vi "Camera Open.vi"(10 "Cluster":T1={"VideoMode"=81, "Brightness"=-1, "Sharpness"=-1, "White Balance"=-1, "Saturation"=-1, "Exposure"=-1} {"VideoMode" items=["640 x 480 YUY 2 30.00 fps", "640 x 480 YUY 2 20.00 fps", "640 x 480 YUY 2 15.00 fps", "640 x 480 YUY 2 10.00 fps", "640 x 480 YUY 2 7.50 fps", "1280 x 720 YUY 2 10.00 fps", "1280 x 720 YUY 2 7.50 fps", "960 x 544 YUY 2 15.00 fps", "960 x 544 YUY 2 10.00 fps", "960 x 544 YUY 2 7.50 fps", "800 x 448 YUY 2 20.00 fps", "800 x 448 YUY 2 15.00 fps", "800 x 448 YUY 2 10.00 fps", "800 x 448 YUY 2 7.50 fps", "640 x 360 YUY 2 30.00 fps", "640 x 360 YUY 2 20.00 fps", "640 x 360 YUY 2 15.00 fps", "640 x 360 YUY 2 10.00 fps", "640 x 360 YUY 2 7.50 fps", "424 x 240 YUY 2 30.00 fps", "424 x 240 YUY 2 20.00 fps", "424 x 240 YUY 2 15.00 fps", "424 x 240 YUY 2 10.00 fps", "424 x 240 YUY 2 7.50 fps", "352 x 288 YUY 2 30.00 fps", "352 x 288 YUY 2 20.00 fps", "352 x 288 YUY 2 15.00 fps", "352 x 288 YUY 2 10.00 fps", "352 x 288 YUY 2 7.50 fps", "320 x 240 YUY 2 30.00 fps", "320 x 240 YUY 2 20.00 fps", "320 x 240 YUY 2 15.00 fps", "320 x 240 YUY 2 10.00 fps", "320 x 240 YUY 2 7.50 fps", "800 x 600 YUY 2 15.00 fps", "800 x 600 YUY 2 10.00 fps", "800 x 600 YUY 2 7.50 fps", "176 x 144 YUY 2 30.00 fps", "176 x 144 YUY 2 20.00 fps", "176 x 144 YUY 2 15.00 fps", "176 x 144 YUY 2 10.00 fps", "176 x 144 YUY 2 7.50 fps", "160 x 120 YUY 2 30.00 fps", "160 x 120 YUY 2 20.00 fps", "160 x 120 YUY 2 15.00 fps", "160 x 120 YUY 2 10.00 fps", "160 x 120 YUY 2 7.50 fps", "1280 x 800 YUY 2 10.00 fps", "640 x 480 JPEG 30.00 fps", "640 x 480 JPEG 20.00 fps", "640 x 480 JPEG 15.00 fps", "640 x 480 JPEG 10.00 fps", "640 x 480 JPEG 7.50 fps", "1280 x 720 JPEG 30.00 fps", "1280 x 720 JPEG 20.00 fps", "1280 x 720 JPEG 15.00 fps", "1280 x 720 JPEG 10.00 fps", "1280 x 720 JPEG 7.50 fps", "960 x 544 JPEG 30.00 fps", "960 x 544 JPEG 20.00 fps", "960 x 544 JPEG 15.00 fps", "960 x 544 JPEG 10.00 fps", "960 x 544 JPEG 7.50 fps", "800 x 448 JPEG 30.00 fps", "800 x 448 JPEG 20.00 fps", "800 x 448 JPEG 15.00 fps", "800 x 448 JPEG 10.00 fps", "800 x 448 JPEG 7.50 fps", "640 x 360 JPEG 30.00 fps", "640 x 360 JPEG 20.00 fps", "640 x 360 JPEG 15.00 fps", "640 x 360 JPEG 10.00 fps", "640 x 360 JPEG 7.50 fps", "800 x 600 JPEG 30.00 fps", "800 x 600 JPEG 20.00 fps", "800 x 600 JPEG 15.00 fps", "800 x 600 JPEG 10.00 fps", "800 x 600 JPEG 7.50 fps", "416 x 240 JPEG 30.00 fps", "416 x 240 JPEG 20.00 fps", "416 x 240 JPEG 15.00 fps", "416 x 240 JPEG 10.00 fps", "416 x 240 JPEG 7.50 fps", "352 x 288 JPEG 30.00 fps", "352 x 288 JPEG 20.00 fps", "352 x 288 JPEG 15.00 fps", "352 x 288 JPEG 10.00 fps", "352 x 288 JPEG 7.50 fps", "176 x 144 JPEG 30.00 fps", "176 x 144 JPEG 20.00 fps", "176 x 144 JPEG 15.00 fps", "176 x 144 JPEG 10.00 fps", "176 x 144 JPEG 7.50 fps", "320 x 240 JPEG 30.00 fps", "320 x 240 JPEG 20.00 fps", "320 x 240 JPEG 15.00 fps", "320 x 240 JPEG 10.00 fps", "320 x 240 JPEG 7.50 fps", "160 x 120 JPEG 30.00 fps", "160 x 120 JPEG 20.00 fps", "160 x 120 JPEG 15.00 fps", "160 x 120 JPEG 10.00 fps", "160 x 120 JPEG 7.50 fps"]}, 11 "InterfaceName":string) -> (0 "error out":errorcluster, 3 "Cluster":T3 {"Camera Settings"."VideoMode" items=["640 x 480 YUY 2 30.00 fps", "640 x 480 YUY 2 20.00 fps", "640 x 480 YUY 2 15.00 fps", "640 x 480 YUY 2 10.00 fps", "640 x 480 YUY 2 7.50 fps", "1280 x 720 YUY 2 10.00 fps", "1280 x 720 YUY 2 7.50 fps", "960 x 544 YUY 2 15.00 fps", "960 x 544 YUY 2 10.00 fps", "960 x 544 YUY 2 7.50 fps", "800 x 448 YUY 2 20.00 fps", "800 x 448 YUY 2 15.00 fps", "800 x 448 YUY 2 10.00 fps", "800 x 448 YUY 2 7.50 fps", "640 x 360 YUY 2 30.00 fps", "640 x 360 YUY 2 20.00 fps", "640 x 360 YUY 2 15.00 fps", "640 x 360 YUY 2 10.00 fps", "640 x 360 YUY 2 7.50 fps", "424 x 240 YUY 2 30.00 fps", "424 x 240 YUY 2 20.00 fps", "424 x 240 YUY 2 15.00 fps", "424 x 240 YUY 2 10.00 fps", "424 x 240 YUY 2 7.50 fps", "352 x 288 YUY 2 30.00 fps", "352 x 288 YUY 2 20.00 fps", "352 x 288 YUY 2 15.00 fps", "352 x 288 YUY 2 10.00 fps", "352 x 288 YUY 2 7.50 fps", "320 x 240 YUY 2 30.00 fps", "320 x 240 YUY 2 20.00 fps", "320 x 240 YUY 2 15.00 fps", "320 x 240 YUY 2 10.00 fps", "320 x 240 YUY 2 7.50 fps", "800 x 600 YUY 2 15.00 fps", "800 x 600 YUY 2 10.00 fps", "800 x 600 YUY 2 7.50 fps", "176 x 144 YUY 2 30.00 fps", "176 x 144 YUY 2 20.00 fps", "176 x 144 YUY 2 15.00 fps", "176 x 144 YUY 2 10.00 fps", "176 x 144 YUY 2 7.50 fps", "160 x 120 YUY 2 30.00 fps", "160 x 120 YUY 2 20.00 fps", "160 x 120 YUY 2 15.00 fps", "160 x 120 YUY 2 10.00 fps", "160 x 120 YUY 2 7.50 fps", "1280 x 800 YUY 2 10.00 fps", "640 x 480 JPEG 30.00 fps", "640 x 480 JPEG 20.00 fps", "640 x 480 JPEG 15.00 fps", "640 x 480 JPEG 10.00 fps", "640 x 480 JPEG 7.50 fps", "1280 x 720 JPEG 30.00 fps", "1280 x 720 JPEG 20.00 fps", "1280 x 720 JPEG 15.00 fps", "1280 x 720 JPEG 10.00 fps", "1280 x 720 JPEG 7.50 fps", "960 x 544 JPEG 30.00 fps", "960 x 544 JPEG 20.00 fps", "960 x 544 JPEG 15.00 fps", "960 x 544 JPEG 10.00 fps", "960 x 544 JPEG 7.50 fps", "800 x 448 JPEG 30.00 fps", "800 x 448 JPEG 20.00 fps", "800 x 448 JPEG 15.00 fps", "800 x 448 JPEG 10.00 fps", "800 x 448 JPEG 7.50 fps", "640 x 360 JPEG 30.00 fps", "640 x 360 JPEG 20.00 fps", "640 x 360 JPEG 15.00 fps", "640 x 360 JPEG 10.00 fps", "640 x 360 JPEG 7.50 fps", "800 x 600 JPEG 30.00 fps", "800 x 600 JPEG 20.00 fps", "800 x 600 JPEG 15.00 fps", "800 x 600 JPEG 10.00 fps", "800 x 600 JPEG 7.50 fps", "416 x 240 JPEG 30.00 fps", "416 x 240 JPEG 20.00 fps", "416 x 240 JPEG 15.00 fps", "416 x 240 JPEG 10.00 fps", "416 x 240 JPEG 7.50 fps", "352 x 288 JPEG 30.00 fps", "352 x 288 JPEG 20.00 fps", "352 x 288 JPEG 15.00 fps", "352 x 288 JPEG 10.00 fps", "352 x 288 JPEG 7.50 fps", "176 x 144 JPEG 30.00 fps", "176 x 144 JPEG 20.00 fps", "176 x 144 JPEG 15.00 fps", "176 x 144 JPEG 10.00 fps", "176 x 144 JPEG 7.50 fps", "320 x 240 JPEG 30.00 fps", "320 x 240 JPEG 20.00 fps", "320 x 240 JPEG 15.00 fps", "320 x 240 JPEG 10.00 fps", "320 x 240 JPEG 7.50 fps", "160 x 120 JPEG 30.00 fps", "160 x 120 JPEG 20.00 fps", "160 x 120 JPEG 15.00 fps", "160 x 120 JPEG 10.00 fps", "160 x 120 JPEG 7.50 fps"]})   [LabVIEW 2015]
uses:
  Camera Data.ctl
  <vilib>/userdefined/High Color/IMAQdx.ctl
  Camera Settings.ctl
  Support Vision Code/38 Video Mode.ctl
  <vilib>/vision/driver/NI_Vision_Acquisition_Software.lvlib
  <resource>/objmgr/imaqdx.rc
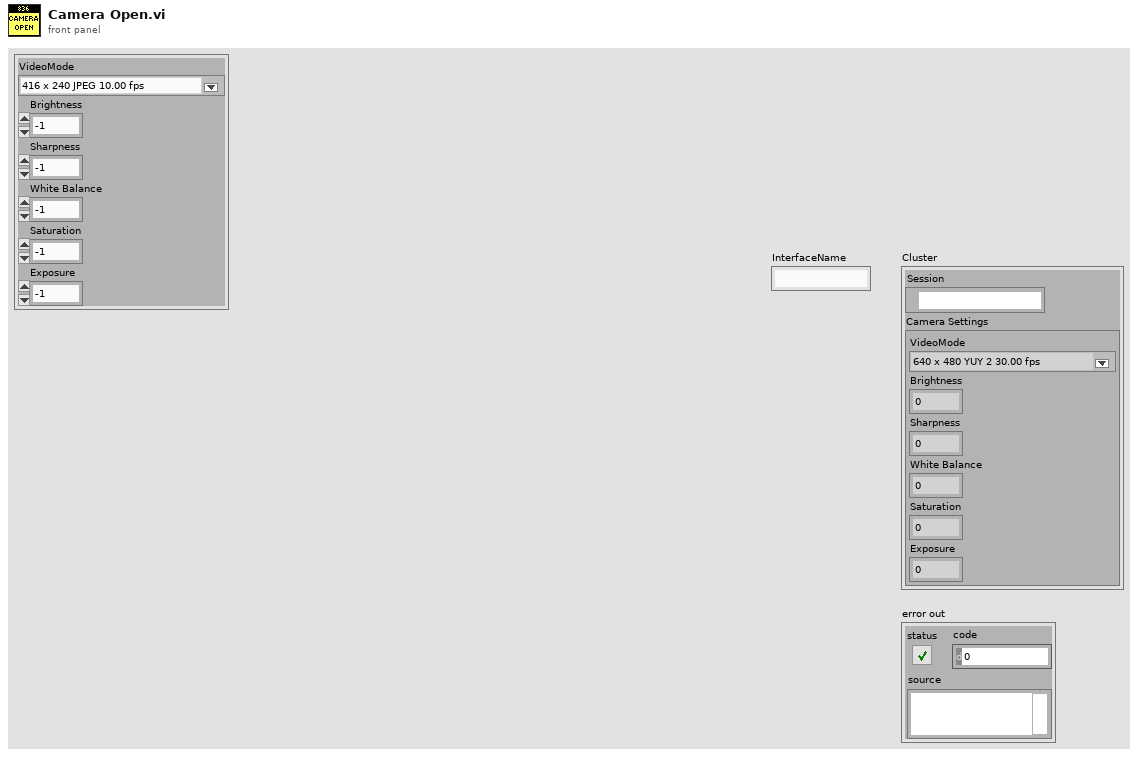
[diagram p1: front panel]
types:
  T1 = typedef "Camera Settings.ctl" = cluster{"VideoMode":T2, "Brightness":i32, "Sharpness":i32, "White Balance":i32, "Saturation":i32, "Exposure":i32}
  T2 = typedef "38 Video Mode.ctl" = u32
  T3 = typedef "Camera Data.ctl" = cluster{"Session":T4, "Camera Settings":T1}
  T4 = typedef "IMAQdx.ctl" = refnum<k21>
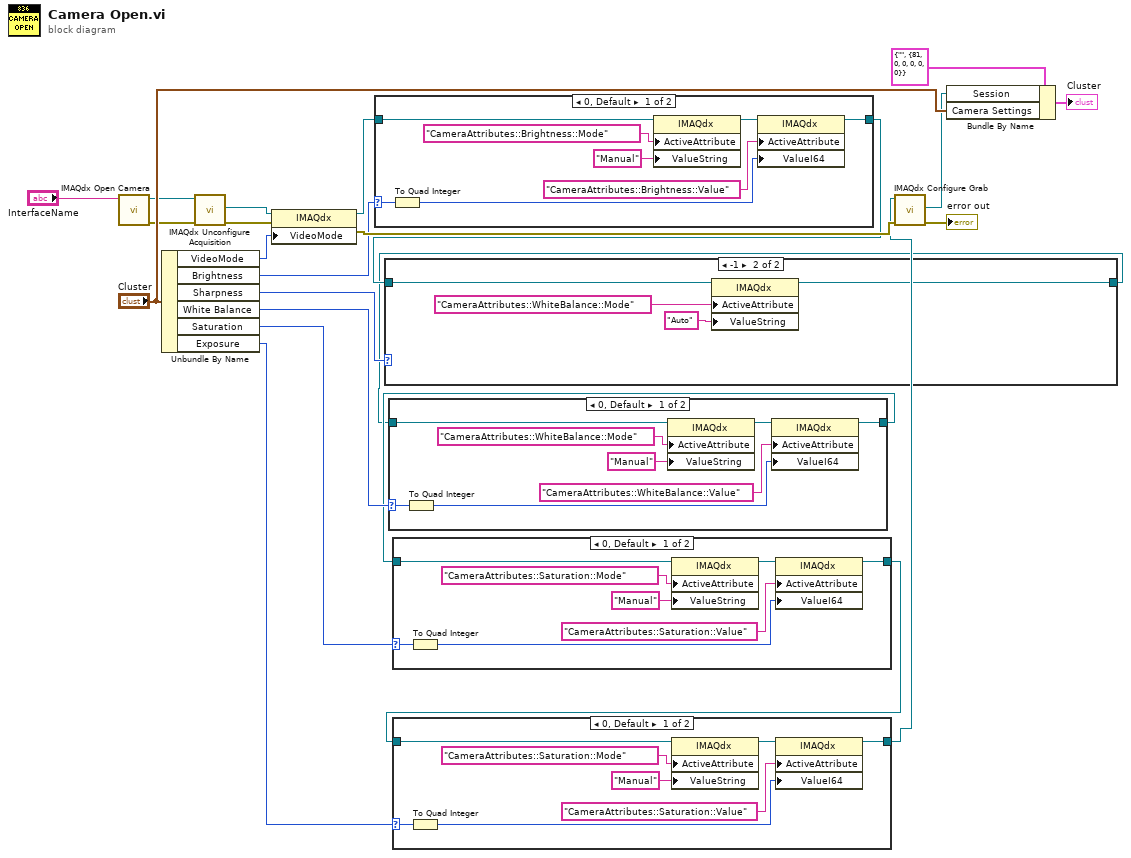
[diagram p0: block diagram]
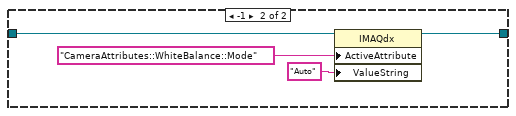
[diagram p2: hidden frame]
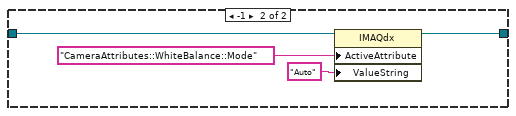
[diagram p3: hidden frame]
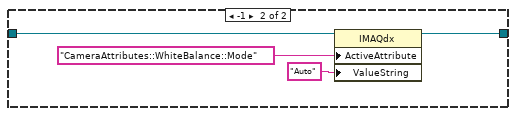
[diagram p4: hidden frame]
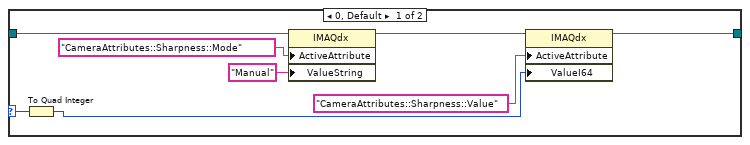
[diagram p5: hidden frame]
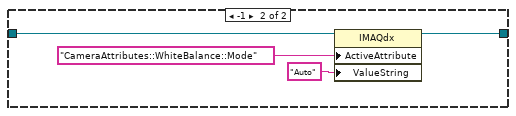
[diagram p6: hidden frame]
diagram:
  n1 = call <vilib>:"IMAQdx Open Camera.vi"("Session In"="InterfaceName") -> ("error out"=w16:errorcluster, "Session Out"=w15:T4)  [unwired: 9 in]
  n2 = Unbundle By Name("Cluster") -> ("VideoMode"=w22:T2, "Brightness"=w11:i32, "Sharpness"=w8:i32, "White Balance"=w7:i32, "Saturation"=w5:i32, "Exposure"=w3:i32)
  n3 = call <vilib>:"IMAQdx Unconfigure Acquisition.vi"("error in"=w16, "Session In"=w15) -> ("error out"=w14:errorcluster, "Session Out"=w13:T4)  [unwired: 8 in]
  n4 = property class="IMAQdx"(reference=w13, error in=w14, "VideoMode"=w22) -> (reference out=w10:T4, error out=w17:errorcluster)
  n5 = case shown="0, Default" w11 {
    selector: w11 -> [w25 _]
    tunnel: w10 -> [w29 w34]
    tunnel: [w27 w32] -> w9
    frame 0, Default {
      n6 = To Quad Integer(1:w25) -> (0:w24:i64)
      n7 = property class="IMAQdx"(reference=w29, "ActiveAttribute"="CameraAttributes::Brightness::Mode", "ValueString"="Manual") -> (reference out=w28:T4)  [unwired: 1 in, 1 out]
      n8 = property class="IMAQdx"(reference=w28, "ActiveAttribute"="CameraAttributes::Brightness::Value", "ValueI64"=w24) -> (reference out=w27:T4)  [unwired: 1 in, 1 out]
    }
    frame -1 {
      n9 = property class="IMAQdx"(reference=w34, "ActiveAttribute"="CameraAttributes::WhiteBalance::Mode", "ValueString"="Auto") -> (reference out=w32:T4)  [unwired: 1 in, 1 out]
    }
  }
  n10 = case shown="-1" w8 {
    selector: w8 -> [w37 _]
    tunnel: w9 -> [w41 w46]
    tunnel: [w38 w44] -> w1
    frame 0, Default {
      n11 = To Quad Integer(1:w37) -> (0:w36:i64)
      n12 = property class="IMAQdx"(reference=w41, "ActiveAttribute"="CameraAttributes::Sharpness::Mode", "ValueString"="Manual") -> (reference out=w40:T4)  [unwired: 1 in, 1 out]
      n13 = property class="IMAQdx"(reference=w40, "ActiveAttribute"="CameraAttributes::Sharpness::Value", "ValueI64"=w36) -> (reference out=w38:T4)  [unwired: 1 in, 1 out]
    }
    frame -1 {
      n14 = property class="IMAQdx"(reference=w46, "ActiveAttribute"="CameraAttributes::WhiteBalance::Mode", "ValueString"="Auto") -> (reference out=w44:T4)  [unwired: 1 in, 1 out]
    }
  }
  n15 = case shown="0, Default" w7 {
    selector: w7 -> [w49 _]
    tunnel: w1 -> [w53 w58]
    tunnel: [w51 w56] -> w6
    frame 0, Default {
      n16 = To Quad Integer(1:w49) -> (0:w48:i64)
      n17 = property class="IMAQdx"(reference=w53, "ActiveAttribute"="CameraAttributes::WhiteBalance::Mode", "ValueString"="Manual") -> (reference out=w52:T4)  [unwired: 1 in, 1 out]
      n18 = property class="IMAQdx"(reference=w52, "ActiveAttribute"="CameraAttributes::WhiteBalance::Value", "ValueI64"=w48) -> (reference out=w51:T4)  [unwired: 1 in, 1 out]
    }
    frame -1 {
      n19 = property class="IMAQdx"(reference=w58, "ActiveAttribute"="CameraAttributes::WhiteBalance::Mode", "ValueString"="Auto") -> (reference out=w56:T4)  [unwired: 1 in, 1 out]
    }
  }
  n20 = case shown="0, Default" w5 {
    selector: w5 -> [w61 _]
    tunnel: w6 -> [w65 w70]
    tunnel: [w63 w68] -> w4
    frame 0, Default {
      n21 = To Quad Integer(1:w61) -> (0:w60:i64)
      n22 = property class="IMAQdx"(reference=w65, "ActiveAttribute"="CameraAttributes::Saturation::Mode", "ValueString"="Manual") -> (reference out=w64:T4)  [unwired: 1 in, 1 out]
      n23 = property class="IMAQdx"(reference=w64, "ActiveAttribute"="CameraAttributes::Saturation::Value", "ValueI64"=w60) -> (reference out=w63:T4)  [unwired: 1 in, 1 out]
    }
    frame -1 {
      n24 = property class="IMAQdx"(reference=w70, "ActiveAttribute"="CameraAttributes::WhiteBalance::Mode", "ValueString"="Auto") -> (reference out=w68:T4)  [unwired: 1 in, 1 out]
    }
  }
  n25 = case shown="0, Default" w3 {
    selector: w3 -> [w73 _]
    tunnel: w4 -> [w77 w82]
    tunnel: [w75 w80] -> w2
    frame 0, Default {
      n26 = To Quad Integer(1:w73) -> (0:w72:i64)
      n27 = property class="IMAQdx"(reference=w77, "ActiveAttribute"="CameraAttributes::Saturation::Mode", "ValueString"="Manual") -> (reference out=w76:T4)  [unwired: 1 in, 1 out]
      n28 = property class="IMAQdx"(reference=w76, "ActiveAttribute"="CameraAttributes::Saturation::Value", "ValueI64"=w72) -> (reference out=w75:T4)  [unwired: 1 in, 1 out]
    }
    frame -1 {
      n29 = property class="IMAQdx"(reference=w82, "ActiveAttribute"="CameraAttributes::WhiteBalance::Mode", "ValueString"="Auto") -> (reference out=w80:T4)  [unwired: 1 in, 1 out]
    }
  }
  n30 = call <vilib>:"IMAQdx Configure Grab.vi"("error in"=w17, "Session In"=w2) -> ("error out"=→"error out":errorcluster, "Session Out"=w20:T4)  [unwired: 8 in]
  n31 = Bundle By Name(cluster=T3 {"Session"="", "Camera Settings"={"VideoMode"=81, "Brightness"=0, "Sharpness"=0, "White Balance"=0, "Saturation"=0, "Exposure"=0}}, "Session"=w20, "Camera Settings"="Cluster") -> (→"Cluster":T3)
